vi "SSL Detection Frame.vi"(8 "error in":errorcluster, 9 "Array":u8[](array[numeric]) format="%02x") -> (0 "error out":errorcluster, 3 "Detection Frame":T1 {"robots_blue"."height" format="%+4.3f"; "robots_blue"."pixel_y" format="%+4.3f"; "robots_blue"."pixel_x" format="%+4.3f"; "robots_blue"."orientation" format="%+4.3f"; "robots_blue"."y" format="%+4.3f"; "robots_blue"."confidence" format="%4.3f"; "robots_blue"."x" format="%+4.3f"; "robots_yellow"."height" format="%+4.3f"; "robots_yellow"."pixel_y" format="%+4.3f"; "robots_yellow"."pixel_x" format="%+4.3f"; "robots_yellow"."orientation" format="%+4.3f"; "robots_yellow"."y" format="%+4.3f"; "robots_yellow"."confidence" format="%4.3f"; "robots_yellow"."x" format="%+4.3f"})   [LabVIEW 2017]
uses:
  Varint Decoder uint32.vi
  SSL Detection Robot.ctl
  SSL Detection Ball.ctl
  SSL Detection Frame.ctl
  <vilib>/Analysis/Matrix/Datatypes/RealMatrix.ctl
  <vilib>/Analysis/Matrix/NI_Matrix.lvlib
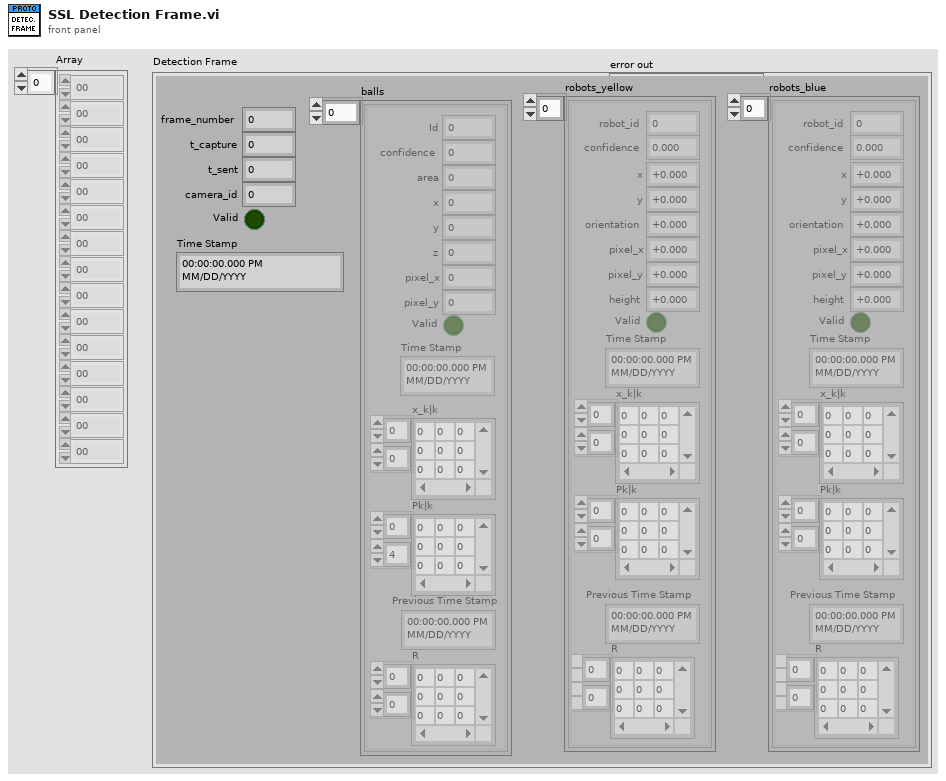
[diagram p1: front panel]
types:
  T1 = typedef "SSL Detection Frame.ctl" = cluster{"frame_number":u32, "t_capture":dbl, "t_sent":dbl, "camera_id":u32, "robots_yellow":T2[], "robots_blue":T2[], "balls":T4[], "Valid":bool, "Time Stamp":timestamp}
  T2 = typedef "SSL Detection Robot.ctl" = cluster{"x":sgl, "robot_id":u32, "confidence":sgl, "y":sgl, "orientation":sgl, "pixel_x":sgl, "pixel_y":sgl, "height":sgl, "Valid":bool, "Time Stamp":timestamp, "x_k|k":T3, "Pk|k":T3, "Previous Time Stamp":timestamp, "R":T3}
  T3 = typedef "NI_Matrix.lvlib/RealMatrix.ctl" = dbl[][]
  T4 = typedef "SSL Detection Ball.ctl" = cluster{"x":sgl, "area":u32, "confidence":sgl, "y":sgl, "z":sgl, "pixel_x":sgl, "pixel_y":sgl, "Valid":bool, "Time Stamp":timestamp, "x_k|k":T3, "Pk|k":T3, "Id":u32, "Previous Time Stamp":timestamp, "R":T3}
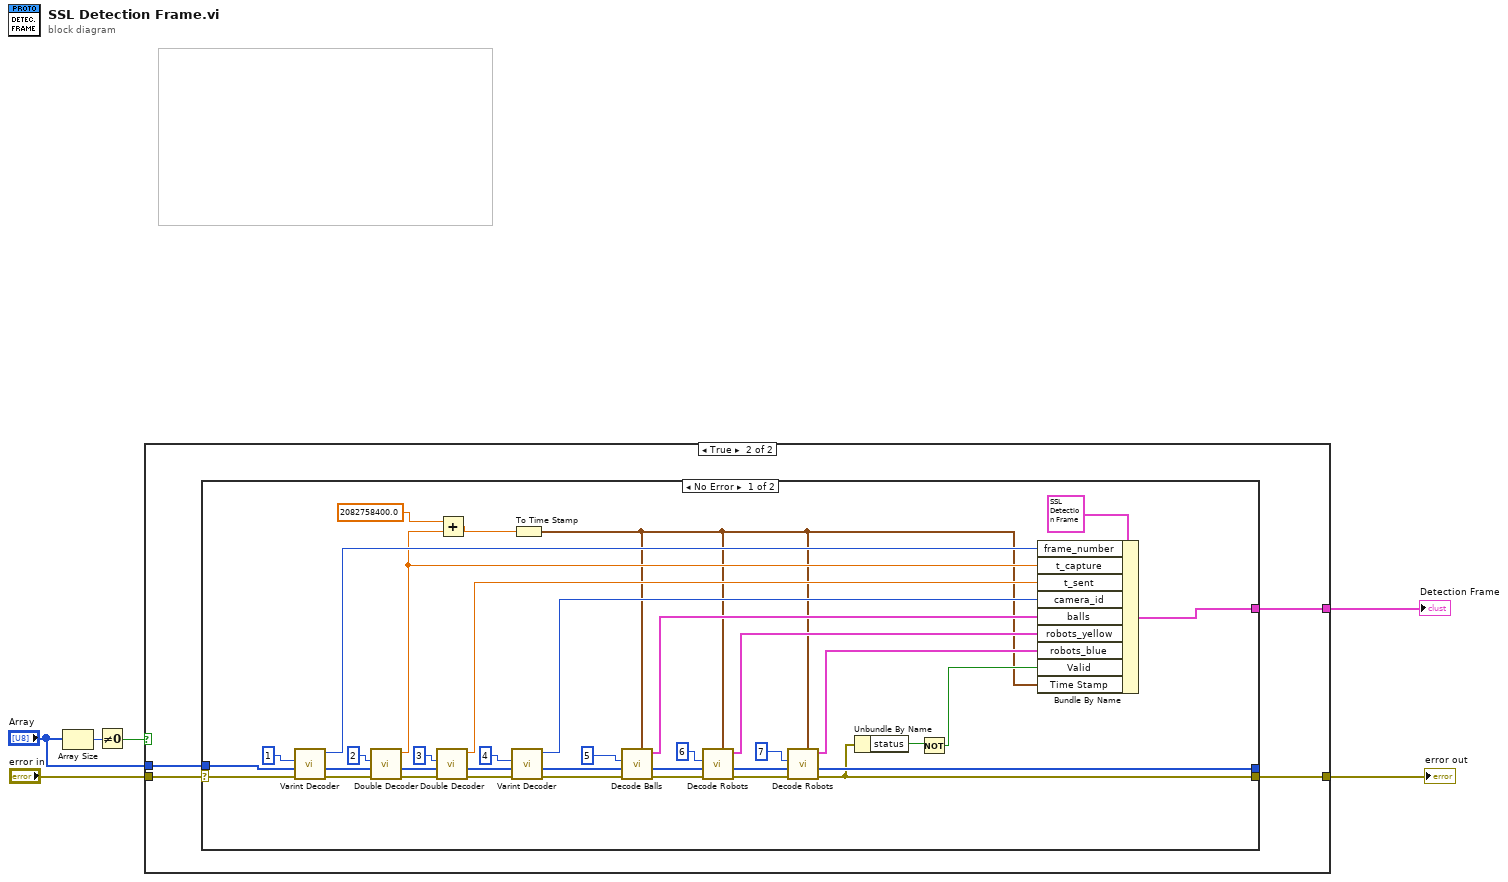
[diagram p0: block diagram]
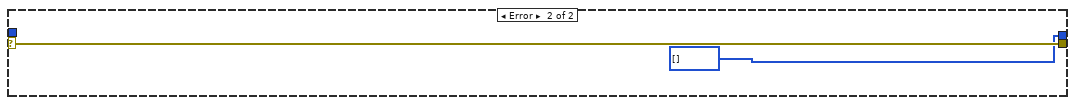
[diagram p3: hidden frame]
diagram:
  n1 = Array Size(array="Array") -> (size(s)=w4:i32)
  n2 = Not Equal To 0?(x=w4) -> (x != 0?=w2:bool)
  n3 = case shown="True" w2 {
    tunnel: "error in" -> [_ w10]
    tunnel: "Array" -> [_ w9]
    tunnel: [_ w8] -> w3
    tunnel: [_ w7] -> w1
    frame False {
    }
    frame True {
      n4 = case shown="No Error" w10 {
        selector: w10 -> [w46 w49]
        tunnel: [w18 w49] -> w8
        tunnel: [w20 u8[] [] ("array w/ subset deleted")] -> _
        tunnel: w9 -> [w19 _]
        tunnel: [w15 _] -> w7
        frame No Error {
          n5 = call-poly "Varint Decoder.vi"("error in (no error)"=w46, "Array"=w19, "Key"=1) -> ("error out"=w45:errorcluster, "array w/ subset deleted"=w30:u8[], "Varint"=w35:u32)  [unwired: 5 in, 1 out]
          n6 = call "Double Decoder.vi"("error in (no error)"=w45, "Array"=w30, "Key"=2) -> ("error out"=w44:errorcluster, "array w/ subset deleted"=w31:u8[], "Double"=w14:dbl)  [unwired: 5 in, 1 out]
          n7 = call "Double Decoder.vi"("error in (no error)"=w44, "Array"=w31, "Key"=3) -> ("error out"=w43:errorcluster, "array w/ subset deleted"=w32:u8[], "Double"=w36:dbl)  [unwired: 5 in, 1 out]
          n8 = Add(x=2082758400.0, y=w14) -> (x+y=w12:dbl)
          n9 = call-poly "Varint Decoder.vi"("error in (no error)"=w43, "Array"=w32, "Key"=4) -> ("error out"=w39:errorcluster, "array w/ subset deleted"=w33:u8[], "Varint"=w37:u32)  [unwired: 5 in, 1 out]
          n10 = To Time Stamp(1:w12) -> (0:w11:timestamp)
          n11 = call "Decode Balls.vi"("Time Stamp"=w11, "error in"=w39, "array"=w33, "Key"=5) -> ("error out"=w28:errorcluster, "array w/ subset deleted out"=w27:u8[], "Array"=w34:T4[])  [unwired: 5 in]
          n12 = call "Decode Robots.vi"("Time Stamp"=w11, "error in"=w28, "array"=w27, "Key"=6) -> ("error out"=w25:errorcluster, "array w/ subset deleted out"=w24:u8[], "Robots"=w22:T2[])  [unwired: 5 in]
          n13 = call "Decode Robots.vi"("Time Stamp"=w11, "error in"=w25, "array"=w24, "Key"=7) -> ("error out"=w18:errorcluster, "array w/ subset deleted out"=w20:u8[], "Robots"=w21:T2[])  [unwired: 5 in]
          n14 = Unbundle By Name(w18) -> ("status"=w17:bool)
          n15 = Not(x=w17) -> (.not. x?=w16:bool)
          n16 = Bundle By Name(cluster=T1 {"frame_number"=0, "t_capture"=0.0, "t_sent"=0.0, "camera_id"=0, "robots_yellow"=[], "robots_blue"=[], "balls"=[], "Valid"=FALSE, "Time Stamp"=timestamp(0 s since 1904-01-01)} ("Detection Frame 2"), "frame_number"=w35, "t_capture"=w14, "t_sent"=w36, "camera_id"=w37, "balls"=w34, "robots_yellow"=w22, "robots_blue"=w21, "Valid"=w16, "Time Stamp"=w11) -> (w15:T1)
        }
        frame Error {
        }
      }
    }
  }
  "error out" <- w3
  "Detection Frame" <- w1
